vi "Is Label Modified.vi"(9 "number of parameters":i32, 10 "initial index":i32, 11 "modified indices":i32[](array[numeric])) -> (2 "label modified":bool)   [LabVIEW 2020, in "Ballard ARINC 429 Engine.lvlib" / "Implementation.lvlib" / "Tx Scheduled Labels Execution Unit.lvclass"]
uses:
  Tx Scheduled Labels Execution Unit.lvclass
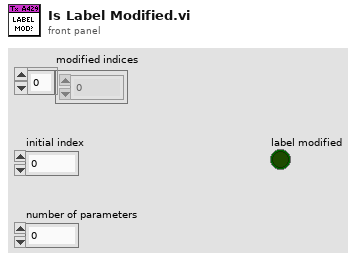
[diagram p1: front panel]
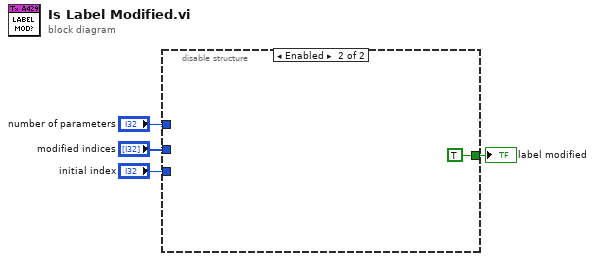
[diagram p0: block diagram]
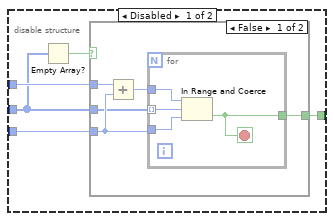
[diagram p2: hidden frame]
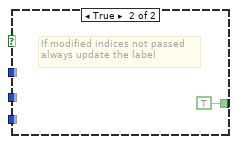
[diagram p3: hidden frame]
diagram:
  n1 = disable-structure shown="Enabled" {
    disable-tunnel: "initial index" -> [w9 _]
    disable-tunnel: "number of parameters" -> [w8 _]
    disable-tunnel: "modified indices" -> [w7 _]
    disable-tunnel: [w5 TRUE ("label modified")] -> w1
    frame Disabled {
      n2 = Empty Array?(array=w7) -> (empty?=w6:bool)
      n3 = case shown="False" w6 {
        tunnel: w9 -> [w13 _]
        tunnel: [w12 TRUE] -> w5
        tunnel: w8 -> [w11 _]
        tunnel: w7 -> [w10 _]
        frame False {
          n4 = Add(x=w11, y=w13) -> (x+y=w14:i32)
          n5 = for {
            tunnel: w10 -> [w18] mode=indexing
            tunnel: w14 -> [w17]
            tunnel: w13 -> [w16]
            tunnel: [w15] -> w12
            stop <- w15 stop-if-true
            n6 = In Range and Coerce(upper limit=w17, x=w18, lower limit=w16) -> (In Range?=w15:bool)  [unwired: 1 out]
          }
        }
        frame True {
          # "If modified indices not passed\nalways update the label"
        }
      }
    }
    frame Enabled {
    }
  }
  "label modified" <- w1
